vi "Nudge Position Down.vi"(8 "error in (no error)":errorcluster, 11 "MulticolumnListbox in":refnum<vi>) -> (0 "error out":errorcluster)   [LabVIEW 2017, in "ListboxExtensions.lvlib"]
uses:
  ListboxExtensions.lvlib
  <vilib>/Utility/miscctls.llb/LVRowAndColumnUnsignedTypeDef.ctl
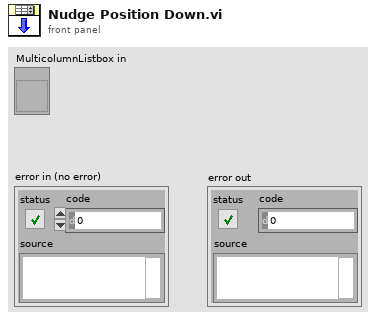
[diagram p1: front panel]
types:
  T1 = typedef "LVRowAndColumnUnsignedTypeDef.ctl" = cluster{"Row":u32, "Column":u32}
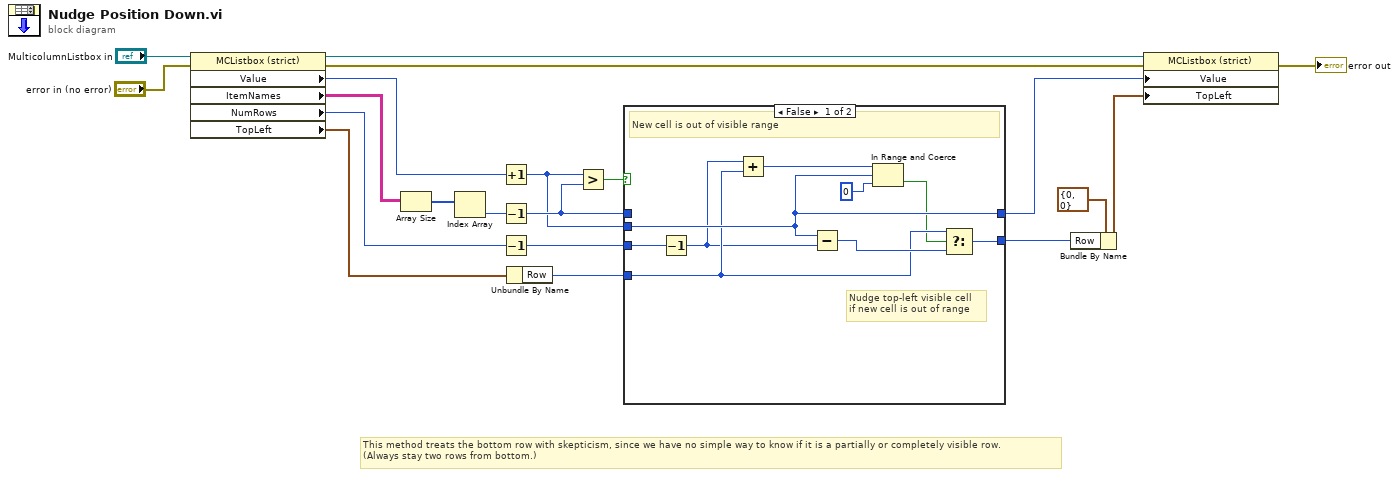
[diagram p0: block diagram]
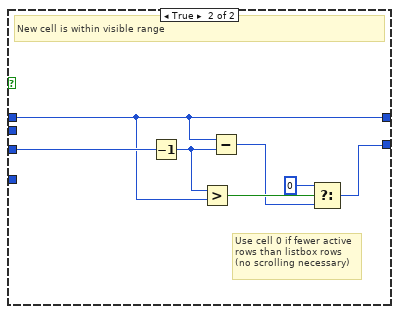
[diagram p2: hidden frame]
diagram:
  # "This method treats the bottom row with skepticism, since we have no simple way to know if it is a partially or completely visible row.\n(Always stay two rows from bottom.)"
  n1 = property class="MCListbox (strict)"(reference="MulticolumnListbox in", error in="error in (no error)") -> (reference out=w10:refnum<vi>, error out=w9:errorcluster, "Value"=w8:i32, "ItemNames"=w6:string[][], "NumRows"=w18:u32, "TopLeft"=w17:T1)
  n2 = Array Size(array=w6) -> (size(s)=w5:i32[])
  n3 = Index Array(array=w5) -> (element=w4:i32)  [unwired: 1 in]
  n4 = Increment(x=w8) -> (x+1=w15:i32)
  n5 = Decrement(x=w4) -> (x-1=w16:i32)
  n6 = Decrement(x=w18) -> (x-1=w19:u32)
  n7 = Unbundle By Name(w17) -> ("Row"=w20:u32)
  n8 = Greater?(x=w15, y=w16) -> (0:w12:bool)
  n9 = case shown="False" w12 {
    tunnel: [w24 w34] -> w13
    tunnel: [w29 w30] -> w14
    tunnel: w20 -> [w23 _]
    tunnel: w15 -> [w24 _]
    tunnel: w19 -> [w26 w36]
    tunnel: w16 -> [_ w34]
    frame False {
      # "Nudge top-left visible cell\nif new cell is out of range"
      # "New cell is out of visible range"
      n10 = Decrement(x=w26) -> (x-1=w22:u32)
      n11 = Add(x=w22, y=w23) -> (x+y=w27:u32)
      n12 = Subtract(x=w24, y=w22) -> (x-y=w25:u32)
      n13 = In Range and Coerce(upper limit=w27, x=w24, lower limit=0) -> (In Range?=w21:bool)  [unwired: 1 out]
      n14 = Select(t=w23, s=w21, f=w25) -> (s? t:f=w29:u32)
    }
    frame True {
      # "Use cell 0 if fewer active\nrows than listbox rows\n(no scrolling necessary)"
      # "New cell is within visible range"
      n15 = Decrement(x=w36) -> (x-1=w35:u32)
      n16 = Greater?(x=w35, y=w34) -> (0:w33:bool)
      n17 = Subtract(x=w34, y=w35) -> (x-y=w31:u32)
      n18 = Select(t=u32 0, s=w33, f=w31) -> (s? t:f=w30:u32)
    }
  }
  n19 = Bundle By Name(cluster=T1 {"Row"=0, "Column"=0} ("Top Left Visible Cell"), "Row"=w14) -> (w2:T1)
  n20 = property class="MCListbox (strict)"(reference=w10, error in=w9, "Value"=w13, "TopLeft"=w2) -> (error out=→"error out":errorcluster)  [unwired: 1 out]
